vi "niDTS WLAN INSTR RX Configure PortManagement.vi"(8 "error in (no error)":errorcluster, 11 "niDTS WLAN INSTR RX in":refnum<class "niDTS WLAN INSTR RX.lvclass">) -> (0 "error out":errorcluster, 3 "niDTS WLAN INSTR RX out":refnum<class "niDTS WLAN INSTR RX.lvclass">)   [LabVIEW 2015, in "niDTS WLAN.lvlib" / "niDTS WLAN INSTR RX.lvclass"]
uses:
  niDTS WLAN INSTR RX.lvclass
  niDTS WLAN INSTR RX.lvclass/niDTS WLAN INSTR RX.ctl
  RiviInstDriver/niRfsgWlan/Objects/niRfsgWlan.lvclass
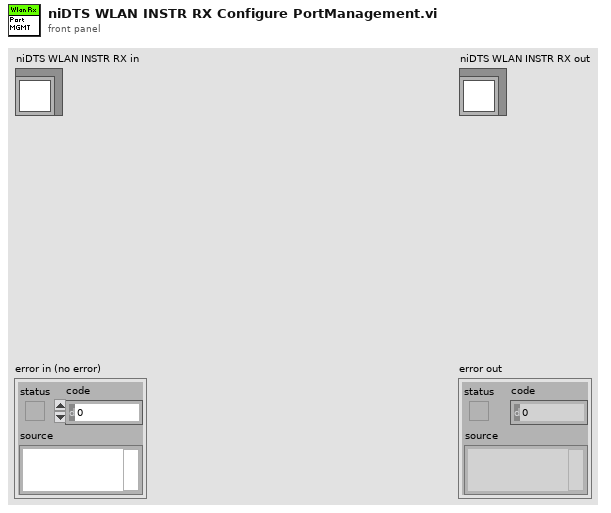
[diagram p1: front panel]
types:
  T1 = typedef "niRfsgWlan.lvclass/niRfsgWlan INC Handle.ctl" = refnum<data-value>
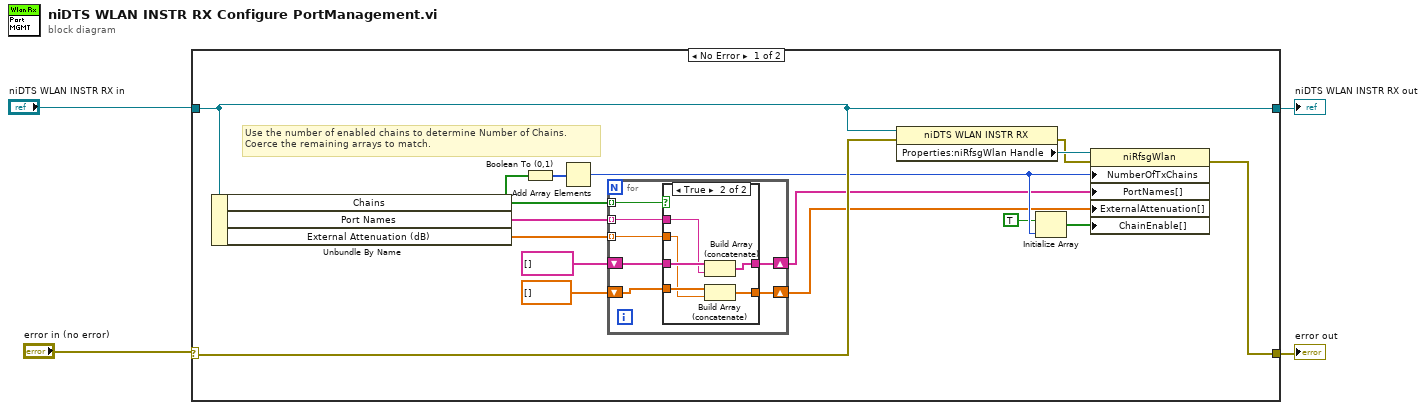
[diagram p0: block diagram]
diagram:
  n1 = case shown="No Error" "error in (no error)" {
    selector: "error in (no error)" -> [w20 w37]
    tunnel: [w17 w37] -> w2
    tunnel: [w5 w36] -> w1
    tunnel: "niDTS WLAN INSTR RX in" -> [w5 w36]
    frame No Error {
      # "Use the number of enabled chains to determine Number of Chains.\nCoerce the remaining arrays to match."
      n2 = Unbundle By Name(w5) -> ("Chains"=w15:bool[], "Port Names"=w14:string[], "External Attenuation (dB)"=w13:dbl[])
      n3 = Boolean To (0,1)(Boolean=w15) -> (0, 1=w16:i16[])
      n4 = Add Array Elements(numeric array=w16) -> (sum=w10:i16)
      n5 = for {
        tunnel: w15 -> [w27] mode=indexing
        tunnel: w14 -> [w21] mode=indexing
        tunnel: w13 -> [w26] mode=indexing
        shift-right: [w23] -> w7
        shift-left: string[] [] ("Port Names") -> [w25]
        shift-right: [w22] -> w6
        shift-left: dbl[] [] ("WLAN Tx Input Parameters.External Attenuation") -> [w24]
        n6 = case shown="True" w27 {
          tunnel: w21 -> [_ w32]
          tunnel: w26 -> [_ w33]
          tunnel: w25 -> [w29 w35]
          tunnel: w24 -> [w28 w34]
          tunnel: [w29 w31] -> w23
          tunnel: [w28 w30] -> w22
          frame False {
          }
          frame True {
            n7 = Build Array (concatenate)(w35, w32) -> (w31:string[])
            n8 = Build Array (concatenate)(w34, w33) -> (w30:dbl[])
          }
        }
      }
      n9 = property class="niDTS WLAN INSTR RX"(reference=w5, error in=w20) -> (error out=w18:errorcluster, "Properties:niRfsgWlan Handle"=w19:T1)  [unwired: 1 out]
      n10 = Initialize Array(TRUE, w10) -> (w8:bool[])
      n11 = property class="niRfsgWlan"(reference=w19, error in=w18, "NumberOfTxChains"=w10, "PortNames[]"=w7, "ExternalAttenuation[]"=w6, "ChainEnable[]"=w8) -> (error out=w17:errorcluster)  [unwired: 1 out]
    }
    frame Error {
    }
  }
  "error out" <- w2
  "niDTS WLAN INSTR RX out" <- w1
